vi "FindStern.vi"(11 "Refnum in":T1) -> (0 "Stern found?":bool, 1 "y pixel":i32, 2 "x pixel":i32, 3 "Refnum out":T1(plugin-control))   [LabVIEW 2011]
uses:
  <vilib>/vision/Image Controls.llb/IMAQ Image.ctl
panel:
  out "Angle":sgl
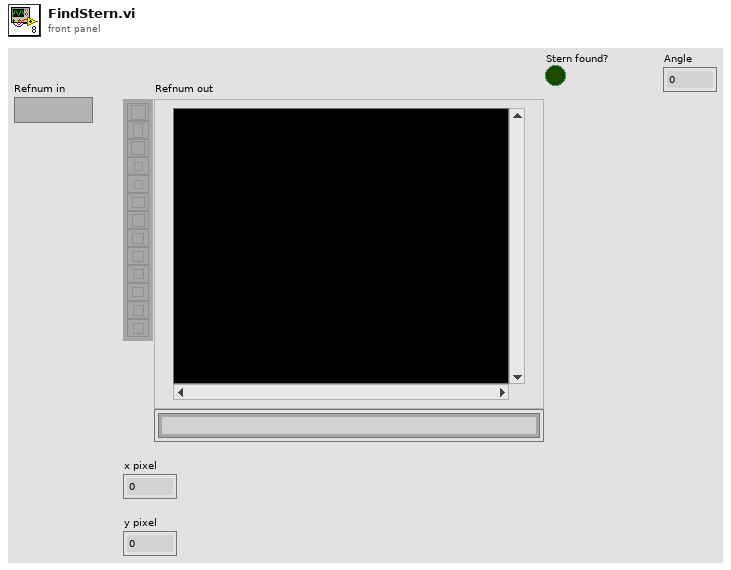
[diagram p1: front panel]
types:
  T1 = typedef "IMAQ Image.ctl" = refnum<image>
  T2 = cluster{"Position":cluster{"x":sgl, "y":sgl}, "Angle":sgl, "Scale":sgl, "Score":sgl, "Bounding Box":cluster{"x":sgl, "y":sgl}[]}[]
  T3 = cluster{"Position":cluster{"x":sgl, "y":sgl}, "Angle":sgl, "Scale":sgl, "Score":sgl, "Bounding Box":cluster{"x":sgl, "y":sgl}[]}
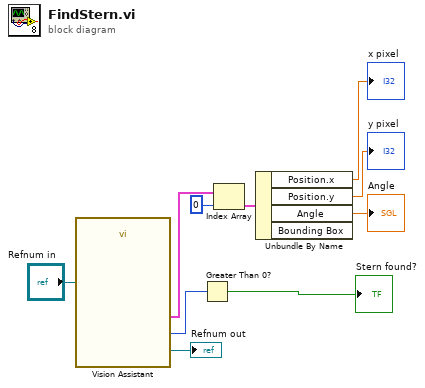
[diagram p0: block diagram]
diagram:
  n1 = call "Vision Assistant"("Image In"="Refnum in") -> ("Image Out"=→"Refnum out":T1, "Matches (Color Pattern Matching 1)"=w7:T2, "Number of Matches (Color Pattern Matching 1)"=w2:i32)  [unwired: 23 in, 1 out]
  n2 = Greater Than 0?(x=w2) -> (x > 0?=→"Stern found?":bool)
  n3 = Index Array(array=w7, index=0) -> (element=w6:T3)
  n4 = Unbundle By Name(w6) -> ("Position.x"=→"x pixel":sgl, "Position.y"=→"y pixel":sgl, "Angle"=→"Angle":sgl)  [unwired: 1 out]
